vi "Set Package Attribute Value.vi"(0 "NI Package Builder solution (.pbs)":path, 5 "package name":string, 7 "package attribute":string, 9 "value":string, 11 "error in (no error)":errorcluster) -> (4 "NI Package Builder solution out":path, 6 "package name out":string, 15 "error out":errorcluster)   [LabVIEW 2017, in "NIPB Solution API.lvlib"]
doc: "Sets the value of the specified attribute of the specified package in the specified NI Package Builder solution (.pbs).\n\nIf the <b>package name</b> input is unwired, this VI will perform this operation on the first package in the NI Package Builder solution and output the corresponding package name in the <b>package name out</b> output."
uses:
  NIPB Solution API.lvlib
  <resource>/objmgr/DOMUserDefRef.rc
  <vilib>/xml/NI_XML.lvlib
  <vilib>/xml/Load XML File.vi
  <vilib>/xml/Close Reference(Node).vi
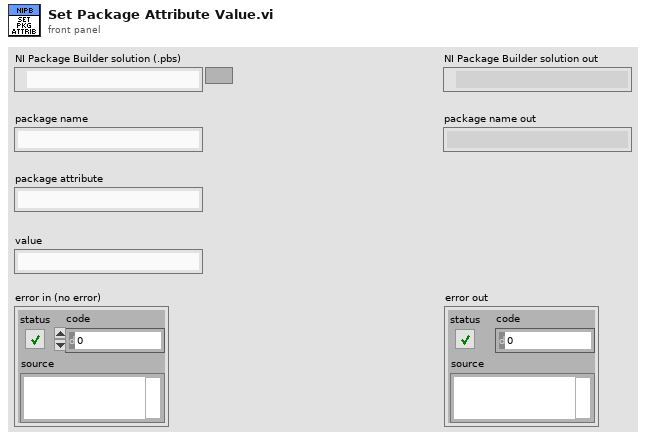
[diagram p1: front panel]
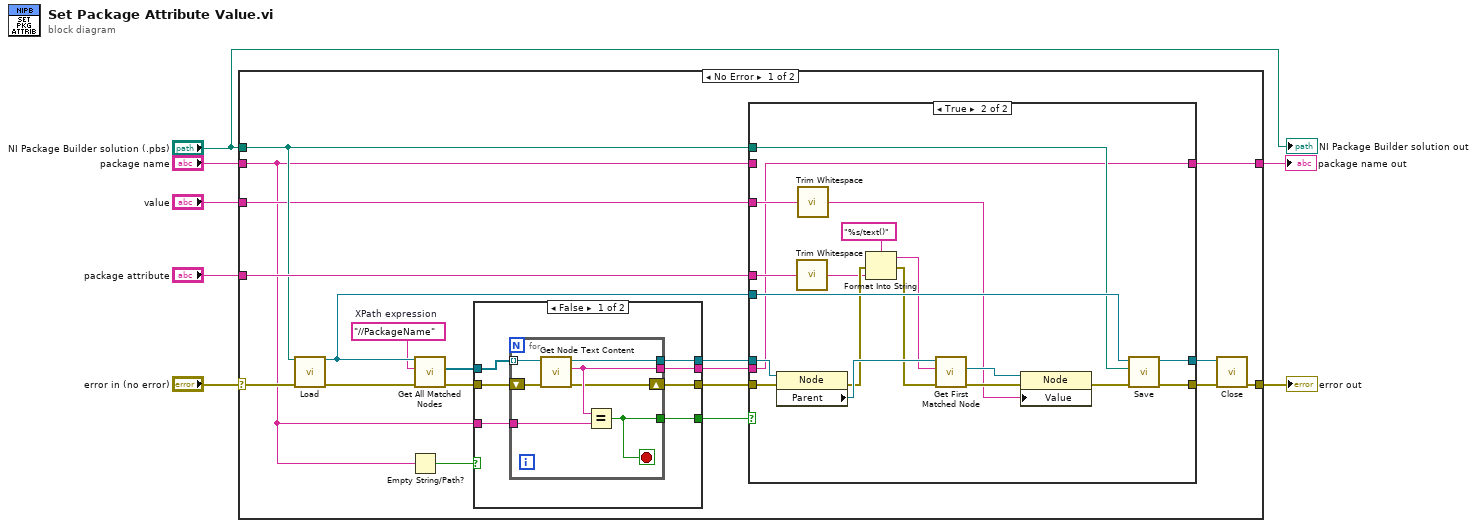
[diagram p0: block diagram]
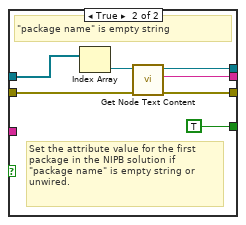
[diagram p2: hidden frame]
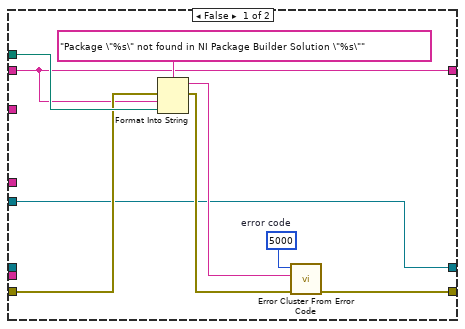
[diagram p3: hidden frame]
diagram:
  n1 = case shown="No Error" "error in (no error)" {
    selector: "error in (no error)" -> [w12 w77]
    tunnel: "package attribute" -> [w26 _]
    tunnel: [w24 w77] -> w6
    tunnel: "package name" -> [w11 w76]
    tunnel: "NI Package Builder solution (.pbs)" -> [w21 _]
    tunnel: "value" -> [w20 _]
    tunnel: [w8 w76] -> w1
    frame No Error {
      w14 = "//PackageName"  # XPath expression
      n2 = call-poly <vilib>:"Load.vi"("path to XML document"=w21, "error in (no error)"=w12) -> ("DOM document out"=w23:refnum<k20>, "error out"=w13:errorcluster)  [unwired: 11 in, 1 out]
      n3 = Empty String/Path?(string/path=w11) -> (empty?=w10:bool)
      n4 = call <vilib>:"Get All Matched Nodes.vi"("error in (no error)"=w13, "XPath expression"=w14, "node in"=w23) -> ("error out"=w16:errorcluster, "node result array"=w15:refnum<k20>[])  [unwired: 6 in, 1 out]
      n5 = case shown="False" w10 {
        tunnel: [w33 w44] -> w19
        tunnel: [w32 w42] -> w18
        tunnel: [w31 TRUE] -> w17
        tunnel: w16 -> [w30 w47]
        tunnel: w15 -> [w29 w46]
        tunnel: w11 -> [w28 _]
        tunnel: [w27 w41] -> w9
        frame False {
          n6 = for {
            tunnel: w29 -> [w37] mode=indexing
            tunnel: [w40] -> w27
            tunnel: w28 -> [w39]
            tunnel: [w38] -> w31
            tunnel: [w34] -> w32
            shift-right: [w35] -> w33
            shift-left: w30 -> [w36]
            stop <- w38 stop-if-true
            n7 = call <vilib>:"Get Node Text Content.vi"("error in (no error)"=w36, "node in"=w37) -> ("error out"=w35:errorcluster, "node text"=w40:string, "node out"=w34:refnum<k20>)  [unwired: 7 in]
            n8 = Equal?(x=w40, y=w39) -> (x = y?=w38:bool)
          }
        }
        frame True {
          # "Set the attribute value for the first package in the NIPB solution if \"package name\" is empty string or unwired."
          # "\"package name\" is empty string"
          n9 = Index Array(array=w46) -> (element=w43:refnum<k20>)  [unwired: 1 in]
          n10 = call <vilib>:"Get Node Text Content.vi"("error in (no error)"=w47, "node in"=w43) -> ("error out"=w44:errorcluster, "node text"=w41:string, "node out"=w42:refnum<k20>)  [unwired: 7 in]
        }
      }
      n11 = case shown="True" w17 {
        tunnel: w18 -> [_ w74]
        tunnel: w19 -> [w52 w73]
        tunnel: w20 -> [_ w71]
        tunnel: w21 -> [w53 w66]
        tunnel: [w56 w67] -> w22
        tunnel: w11 -> [w48 _]
        tunnel: w23 -> [w49 w72]
        tunnel: [w49 w64] -> w25
        tunnel: w26 -> [_ w62]
        tunnel: w9 -> [_ w57]
        tunnel: [w48 w57] -> w8
        frame False {
          w55 = 5000  # error code
          n12 = Format Into String(format string="Package \"%s\" not found in NI Package Builder Solution \"%s\"", error in=w52, w48, w53) -> (resulting string=w50:string, error out=w51:errorcluster)  [unwired: 1 in]
          n13 = call <vilib>:"Error Cluster From Error Code.vi"("error in (no error)"=w51, "error message (\"\")"=w50, "error code (0)"=w55) -> ("error out"=w56:errorcluster)  [unwired: 6 in]
        }
        frame True {
          n14 = property class="Node"(reference=w74, error in=w73) -> (error out=w61:errorcluster, "Parent"=w75:refnum<k20>)  [unwired: 1 out]
          n15 = call <vilib>:"Trim Whitespace.vi"("string"=w62) -> ("trimmed string"=w58:string)  [unwired: 1 in]
          n16 = call <vilib>:"Trim Whitespace.vi"("string"=w71) -> ("trimmed string"=w65:string)  [unwired: 1 in]
          n17 = Format Into String(format string="%s/text()", error in=w61, w58) -> (resulting string=w59:string, error out=w60:errorcluster)  [unwired: 1 in]
          n18 = call <vilib>:"Get First Matched Node.vi"("error in (no error)"=w60, "XPath expression"=w59, "node in"=w75) -> ("error out"=w68:errorcluster, "node result"=w70:refnum<k20>)  [unwired: 6 in, 1 out]
          n19 = property class="Node"(reference=w70, error in=w68, "Value"=w65) -> (error out=w69:errorcluster)  [unwired: 1 out]
          n20 = call <vilib>:"Save.vi"("error in (no error)"=w69, "XML file path"=w66, "DOM document in"=w72) -> ("error out"=w67:errorcluster, "DOM document out"=w64:refnum<k20>)  [unwired: 6 in, 1 out]
        }
      }
      n21 = call-poly <vilib>:"Close.vi"("error in (no error)"=w22, "node"=w25) -> ("error out"=w24:errorcluster)  [unwired: 7 in]
    }
    frame Error {
    }
  }
  "error out" <- w6
  "package name out" <- w1
  "NI Package Builder solution out" <- "NI Package Builder solution (.pbs)"
